vi "OP20 Indicators.vi"(8 "error in (no error)":errorcluster, 10 "Array":refnum<vi>[](array[refnum]), 11 "OUTPUT INDICATOR in":T1) -> (0 "error out":errorcluster, 3 "OUTPUT INDICATOR out":T1)   [LabVIEW 2017]
uses:
  8bcb6a2e-dfd2-4f6b-b5e2-eb446c823387.vi
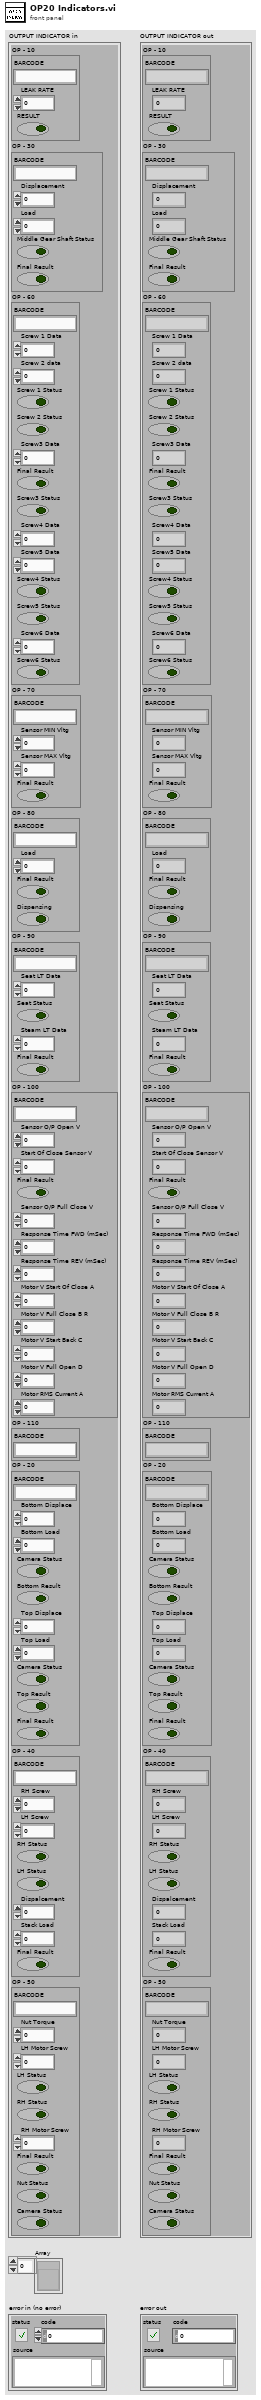
[diagram p1: front panel]
types:
  T1 = cluster{"OP - 10":cluster{"BARCODE":string, "LEAK RATE":dbl, "RESULT":bool}, "OP - 30":cluster{"BARCODE":string, "Displacement":dbl, "Load":dbl, "Middle Gear Shaft Status":bool, "Final Result":bool}, "OP - 60":cluster{"BARCODE":string, "Screw 1 Data":dbl, "Screw 2 data":dbl, "Screw 1 Status":bool, "Screw 2 Status":bool, "Screw3 Data":dbl, "Final Result":bool, "Screw3 Status":bool, "Screw4 Data":dbl, "Screw5 Data":dbl, "Screw4 Status":bool, "Screw5 Status":bool, "Screw6 Data":dbl, "Screw6 Status":bool}, "OP - 70":cluster{"BARCODE":string, "Sensor MIN Vltg":dbl, "Sensor MAX Vltg":dbl, "Final Result":bool}, "OP - 80":cluster{"BARCODE":string, "Load":dbl, "Final Result":bool, "Dispensing":bool}, "OP - 90":cluster{"BARCODE":string, "Seat LT Data":dbl, "Seat Status":bool, "Steam LT Data":dbl, "Final Result":bool}, "OP - 100":cluster{"BARCODE":string, "Sensor O/P Open V":dbl, "Start Of Close Sensor V":dbl, "Final Result":bool, "Sensor O/P Full Close V":dbl, "Response Time FWD (mSec)":dbl, "Response Time REV (mSec)":dbl, "Motor V Start Of Close A":dbl, "Motor V Full Close B R":dbl, "Motor V Start Back C":dbl, "Motor V Full Open D":dbl, "Motor RMS Current A":dbl}, "OP - 110":cluster{"BARCODE":string}, "OP - 20":cluster{"BARCODE":string, "Bottom Displace":dbl, "Bottom Load":dbl, "Camera Status":bool, "Bottom Result":bool, "Top Displace":dbl, "Top Load ":dbl, "Camera Status":bool, "Top Result":bool, "Final Result":bool}, "OP - 40":cluster{"BARCODE":string, "RH Screw":dbl, "LH Screw ":dbl, "RH Status":bool, "LH Status":bool, "Dispalcement ":dbl, "Stack Load ":dbl, "Final Result":bool}, "OP - 50":cluster{"BARCODE":string, "Nut Torque":dbl, "LH Motor Screw":dbl, "LH Status":bool, "RH Status":bool, "RH Motor Screw":dbl, "Final Result":bool, "Nut Status":bool, "Camera Status":bool}}
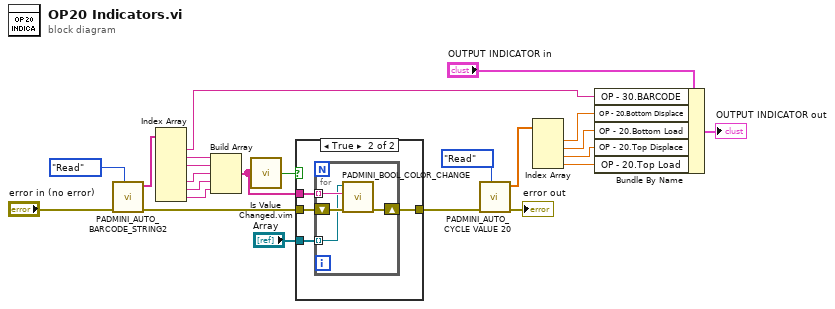
[diagram p0: block diagram]
diagram:
  n1 = call "PADMINI_AUTO_BARCODE_STRING2.vi"("Enum"=enum16{"Read", "Write"}."Read", "error in (no error)"="error in (no error)") -> ("error out"=w5:errorcluster, "Input 2"=w4:string[])  [unwired: 8 in]
  n2 = Index Array(array=w4) -> (element #1=w2:string, element #2=w13:string, element #3=w14:string, element #5=w15:string, element #6=w16:string, element #7=w17:string)  [unwired: 7 in, 1 out]
  n3 = Build Array(w13, w14, w15, w16, w17) -> (w18:string[])
  n4 = call "Is Value Changed.vim"("value"=w18) -> ("changed or first call?"=w1:bool)
  n5 = case shown="True" w1 {
    tunnel: [w24 w28] -> w21
    tunnel: w18 -> [_ w27]
    tunnel: w5 -> [w24 w26]
    tunnel: "Array" -> [_ w25]
    frame False {
    }
    frame True {
      n6 = for {
        tunnel: w27 -> [w31] mode=indexing
        shift-right: [w32] -> w28
        shift-left: w26 -> [w30]
        tunnel: w25 -> [w29] mode=indexing
        n7 = call "PADMINI_BOOL_COLOR_CHANGE.vi"("error in (no error)"=w30, "Input Result"=w31, "Boolean in"=w29) -> ("error out"=w32:errorcluster)  [unwired: 8 in]
      }
    }
  }
  n8 = call "PADMINI_AUTO_CYCLE VALUE 20.vi"("Enum"=enum16{"Read", "Write"}."Read", "error in (no error)"=w21) -> ("error out"=→"error out":errorcluster, "Input 2"=w20:sgl[])  [unwired: 8 in]
  n9 = Index Array(array=w20) -> (element #1=w6:sgl, element #2=w9:sgl, element #3=w10:sgl, element #4=w11:sgl)  [unwired: 4 in]
  n10 = Bundle By Name(cluster="OUTPUT INDICATOR in", "OP - 30.BARCODE"=w2, "OP - 20.Bottom Displace"=w6, "OP - 20.Bottom Load"=w9, "OP - 20.Top Displace"=w10, "OP - 20.Top Load"=w11) -> (→"OUTPUT INDICATOR out":T1)
